vi "Count Stop.vi"(11 "handle":i32) -> (2 "function return":i32, 3 "handle out":i32)   [LabVIEW 2022 SP3]
doc: "BOOL H11890API __stdcall H11890CountStop(HANDLE handle);"
uses:
  H11890api.dll
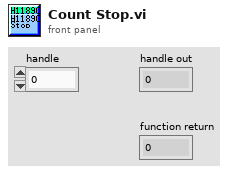
[diagram p1: front panel]
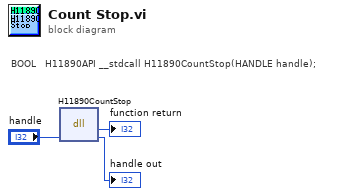
[diagram p0: block diagram]
diagram:
  # "BOOL\t\t\tH11890API __stdcall H11890CountStop(HANDLE handle);"
  n1 = dll-call lib="C:/Users/Public/OneDrive/Desktop/PMT_Project_folder/PMT_VIs/H11890api.dll" fn="H11890CountStop"("handle"="handle") -> ("Return"=→"function return":i32, "handle"=→"handle out":i32)  [unwired: 3 in, 2 out]
